vi "InitDigitizer.vi"(8 "error in":errorcluster, 11 "FPGA VI Reference":T1) -> (0 "error out":errorcluster, 2 "range (Vpp)":dbl=1.3, 3 "FPGA VI Reference Out":T1, 5 "TIS Configured?":bool, 7 "Configured?":bool)   [LabVIEW 2020]
uses:
  DigiFPGARef.ctl
  Controls/TIS Mode.ctl
  Controls/FPGA VI Reference.ctl
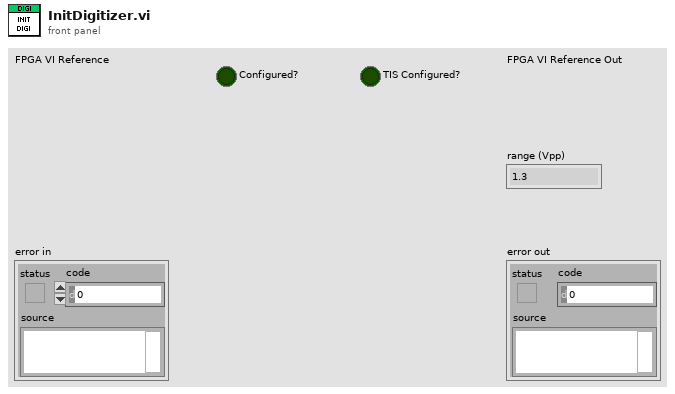
[diagram p1: front panel]
types:
  T1 = typedef "DigiFPGARef.ctl" = refnum<k20>
  T2 = typedef "FPGA VI Reference.ctl" = refnum<k20>
  T3 = typedef "TIS Mode.ctl" = u16
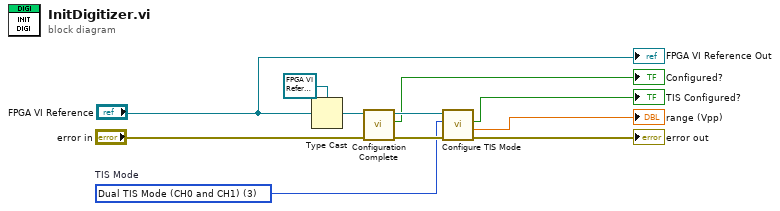
[diagram p0: block diagram]
diagram:
  w7 = T3 3 items=["TIS Mode (CH0 Only)"=1, "TIS Mode (CH1 Only)"=2, "Dual TIS Mode (CH0 and CH1)"=3]  # TIS Mode
  n1 = Type Cast(type=T2 refnum ("FPGA VI Reference In"), x="FPGA VI Reference") -> (*(type *) &x=w4:T2)
  n2 = call "Configuration Complete.vi"("error in"="error in", "FPGA VI Reference In"=w4) -> ("error out"=w11:errorcluster, "Configured?"=→"Configured?":bool, "FPGA VI Reference Out"=w10:T2)  [unwired: 7 out]
  n3 = call "Configure TIS Mode.vi"("error in"=w11, "TIS Mode"=w7, "FPGA VI Reference In"=w10) -> ("error out"=→"error out":errorcluster, "range (Vpp)"=→"range (Vpp)":dbl, "TIS Configured?"=→"TIS Configured?":bool)  [unwired: 5 in, 1 out]
  "FPGA VI Reference Out" <- "FPGA VI Reference"
